vi "Main.vi"() -> ()   [LabVIEW 2015]
doc: "This template is for the Queued Message Handler design pattern.\n\nThe Event Handling Loop generates messages based on user interface actions.\n\nThe Message Handling Loop processes messages generated by the Event Handling Loop, or by other messages. The messages are string values, so new messages can be added easily to the Message Cases case structure in the Message Handling Loop. Each message cluster can also provide an optional value for Message Data, which is a variant that can be converted to whatever message-specific data is required."
uses:
  support/Type Definitions/UI Data.ctl
  support/Status Logger/Status Log.ctl
  <vilib>/Utility/error.llb/DialogType.ctl
  DAQ/TypeDefs/DAQ data.ctl
  support/Message Queue/Enqueue Message (Single).vi
  support/Global names.vi
  <vilib>/Utility/error.llb/Error Cluster From Error Code.vi
  <vilib>/ErrorRing/Error Ring.xnode
  support/Message Queue/Message Queue.lvlib
  support/User Event - EHL Stop/User Event - EHL Stop.lvlib
  Model/Model.lvlib
  DAQ/DAQ.lvlib
  PLC/PLC.lvlib
  Logger/Logger.lvlib
panel:
  out "Power status":bool
  in  "Remote":bool
  in  "Abort":bool
  in  "Stop Line":bool
  in  "Start Line":bool
  out "Status":string
  in  "Tab Control":T1(tab)
  in  "Power switch":bool
  in  "Positon":dbl(slide) scale=0.0..20.0
  in  "Dispose":bool
  in  "Pump":bool
  in  "Flow [l/s]":dbl=10.0
  in  "Potentiometer (AI)":tag
  in  "LED (DO)":tag
  in  "Bistable switch (DI)":tag
  in  "Monostable switch (DI)":tag
  in  "Send":bool
  in  "Data to send":string
  out "Data received":string
  in  "Disconnect":bool
  in  "Connect":bool
  out "Connected?":bool
  in  "Type":enum16{"Server", "Client"}(ring)
  in  "Port":u16
  in  "IP":string
  in  "Current printer":u16(ring) items=["PDFCreator", "OKI DATA CORP C5950 kolor (C-2 218)", "Microsoft XPS Document Writer", "Microsoft Print to PDF", "HP LaserJet Professional P1606dn B&W (M3)", "hp LaserJet 1320 PCL 5 B&W (C-2 307)", "Fax", "Canon MP560 KOLOR (DOM)", "Brother PC-FAX v.3.2", "Brother MFC-L8850CDW KOLOR (M6)", "Brother MFC-L2740DW B&W (M6)", "Brother MFC-L2740DW B&W (M3)", "Brother DCP-9020CDW (Dziekan)"]
  in  "Check printers":bool
  in  "Print report":bool
  in  "TDMS View":bool
  in  "Exit":bool
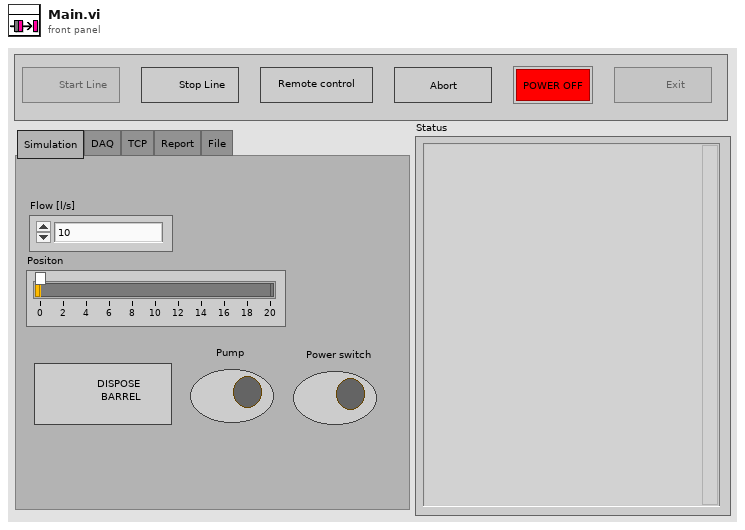
[diagram p1: front panel]
types:
  T1 = enum32{"Simulation", "DAQ", "TCP", "Report", "File"}
  T2 = typedef "Status Log.ctl" = enum16{"Close file", "Open Status file", "Add Status", "Show Status File"}
  T3 = typedef "UI Data.ctl" = cluster{"Start Line Ref":refnum<vi>, "Stop Line Ref":refnum<vi>, "Data Display Ref":refnum<vi>, "Exit Button Ref":refnum<vi>, "Pump Ref":refnum<vi>, "Dispose Ref":refnum<vi>, "Flow Ref":refnum<vi>, "Position Ref":refnum<vi>, "Tab Ref":refnum<vi>, "Print report":refnum<vi>, "Remote":refnum<vi>, "Connection status":refnum<vi>, "Abort":refnum<vi>, "Power status":refnum<vi>, "Power switch":refnum<vi>}
  T4 = typedef "Notifiers.lvlib/Notifiers.ctl" = cluster{"PLC":refnum<notifier>, "Model":refnum<notifier>, "DAQ":refnum<notifier>, "Log":refnum<notifier>}
  T5 = typedef "Message Queue.lvlib/All Message Queues.ctl" = cluster{"UI":refnum<queue>, "Model":refnum<queue>, "DAQ":refnum<queue>, "PLC":refnum<queue>, "Log":refnum<queue>}
  T6 = typedef "DialogType.ctl" = u16
  T7 = typedef "DAQ.lvlib/DAQ data.ctl" = cluster{"Power switch (DI)":cluster{"Channel":tag, "Data":bool}, "Dispose barrel (DI)":cluster{"Channel":tag, "Data":bool}, "Pump status (DO)":cluster{"Channel":tag, "Data":bool}, "Barrel position (AI)":cluster{"Channel":tag, "Data":dbl}}
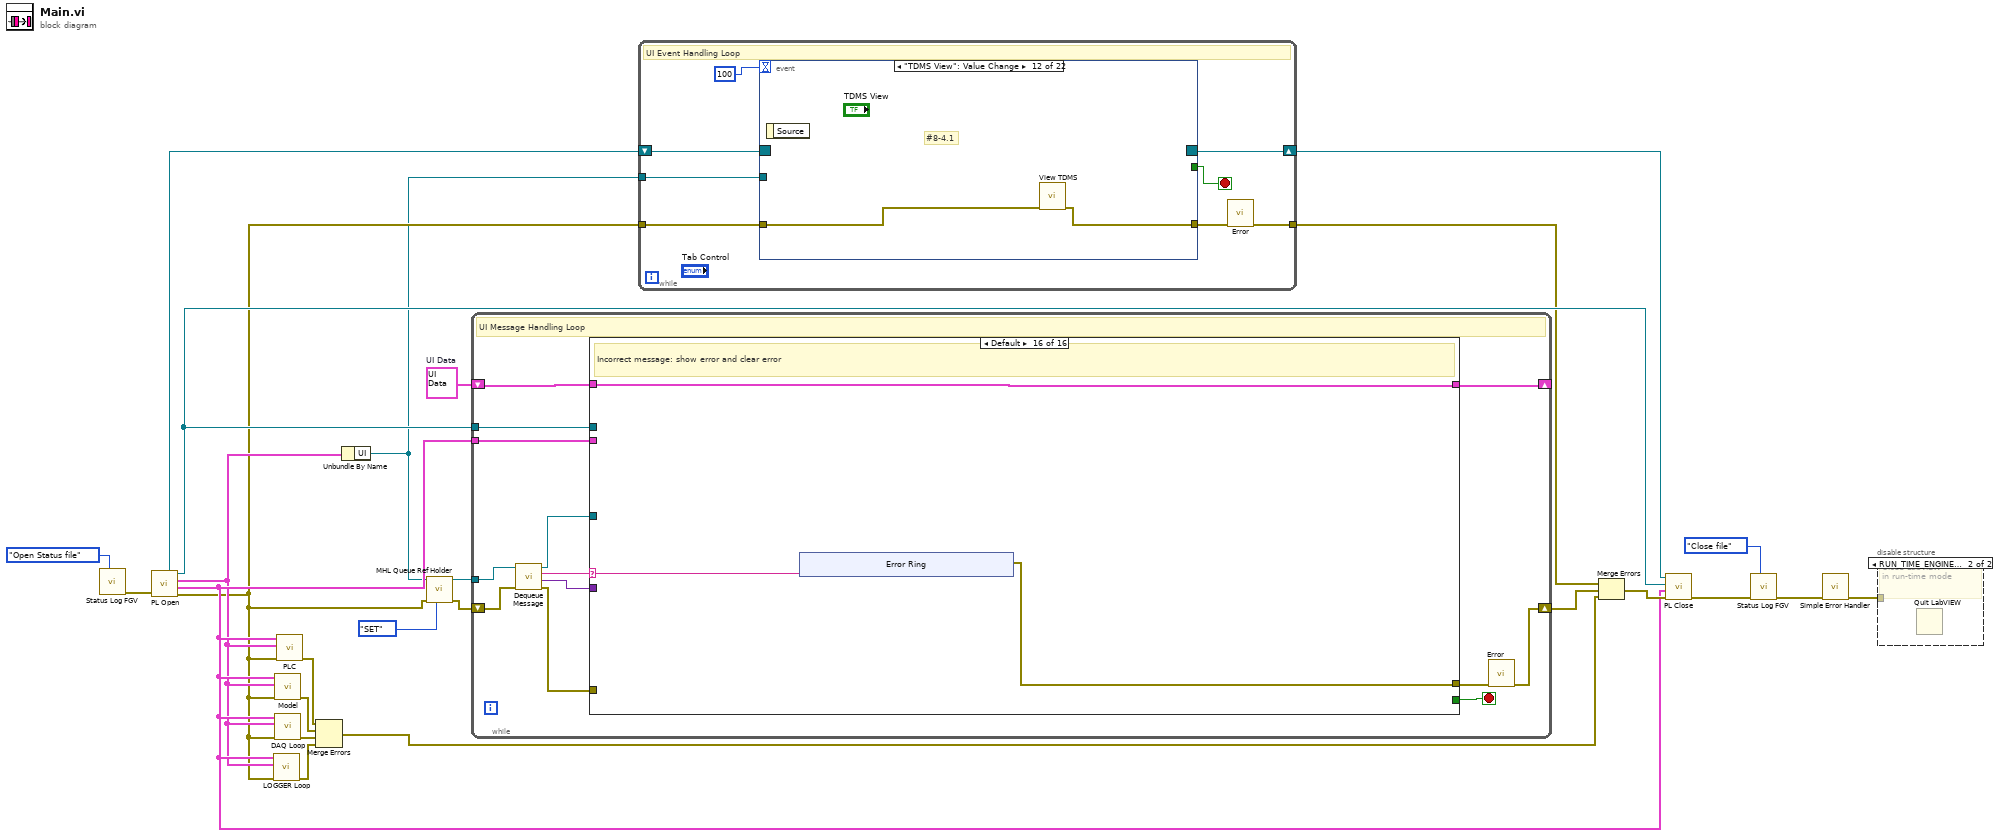
[diagram p0: block diagram]
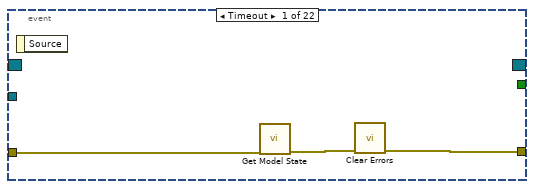
[diagram p2: hidden frame]
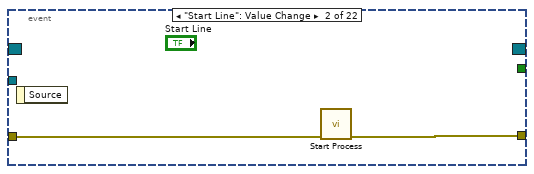
[diagram p3: hidden frame]
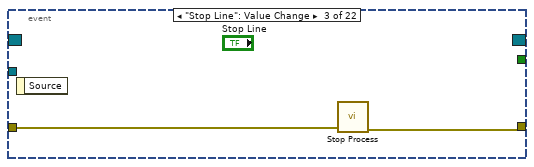
[diagram p4: hidden frame]
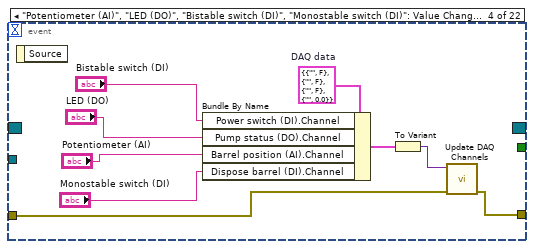
[diagram p5: hidden frame]
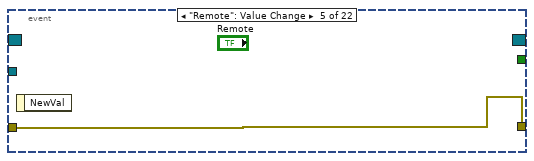
[diagram p6: hidden frame]
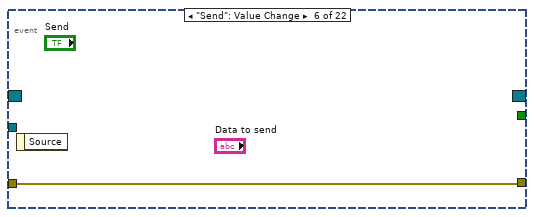
[diagram p7: hidden frame]
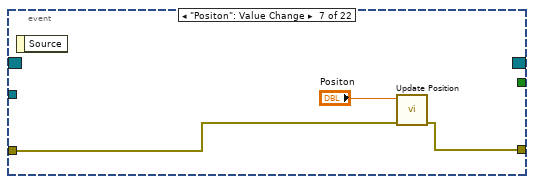
[diagram p8: hidden frame]
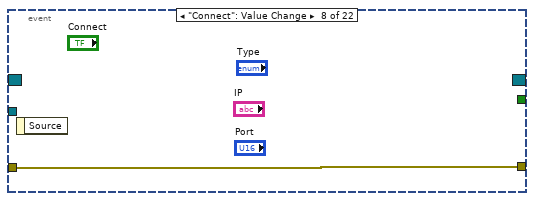
[diagram p9: hidden frame]
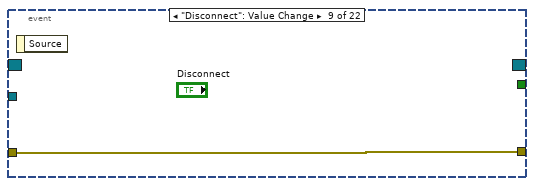
[diagram p10: hidden frame]
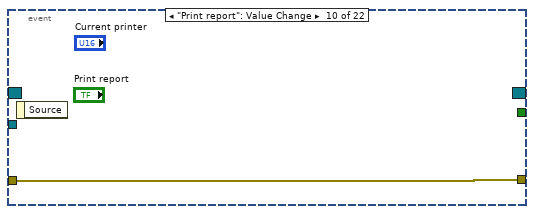
[diagram p11: hidden frame]
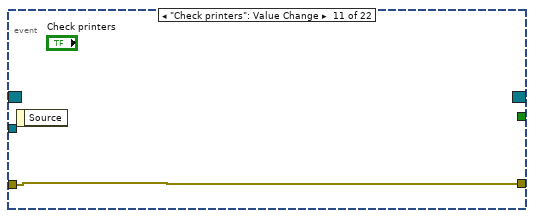
[diagram p12: hidden frame]
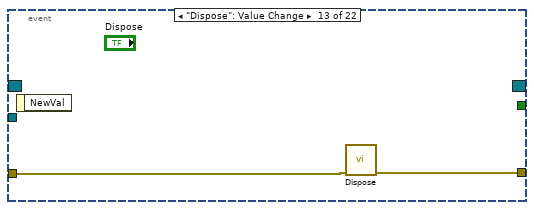
[diagram p13: hidden frame]
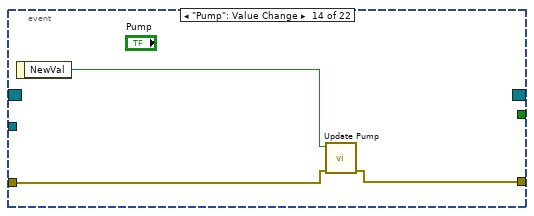
[diagram p14: hidden frame]
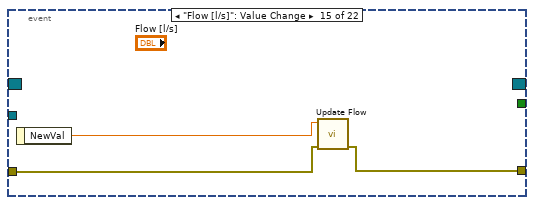
[diagram p15: hidden frame]
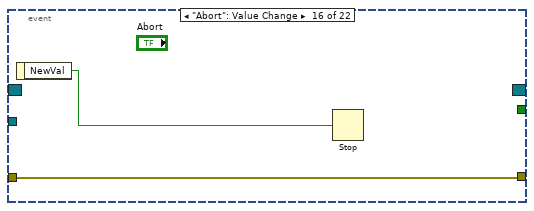
[diagram p16: hidden frame]
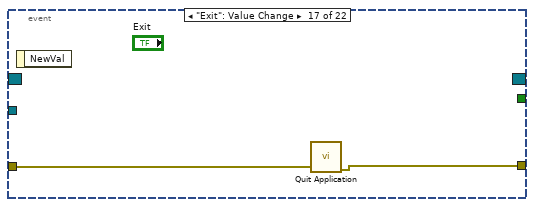
[diagram p17: hidden frame]
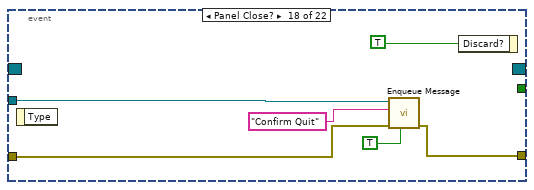
[diagram p18: hidden frame]
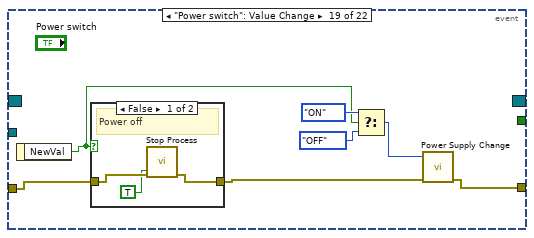
[diagram p19: hidden frame]
diagram:
  w24 = T3 {"Start Line Ref"=refnum, "Stop Line Ref"=refnum, "Data Display Ref"=refnum, "Exit Button Ref"=refnum, "Pump Ref"=refnum, "Dispose Ref"=refnum, "Flow Ref"=refnum, "Position Ref"=refnum, "Tab Ref"=refnum, "Print report"=refnum, "Remote"=refnum, "Connection status"=refnum, "Abort"=refnum, "Power status"=refnum, "Power switch"=refnum}  # UI Data
  n1 = call "Status Log FGV.vi"("Action"=Status_Log."Open Status file") -> ("error out"=w19:errorcluster)  [unwired: 10 in]
  n2 = call "PL Open.vi"("error in"=w19) -> ("error out"=w4:errorcluster, "Notifiers"=w12:T4, "Queues"=w11:T5, "User Event"=w22:refnum<user-event>, "Event Registration Refnum"=w14:refnum<event-registration>)  [unwired: 6 in]
  n3 = call "LOGGER Loop.vi"("error in"=w4, "Queues"=w11, "Notifiers"=w12) -> ("error out"=w7:errorcluster)  [unwired: 8 in]
  n4 = call "Model.vi"("error in"=w4, "Queues"=w11, "Notifiers"=w12) -> ("error out"=w9:errorcluster)  [unwired: 8 in]
  n5 = call "DAQ Loop.vi"("error in"=w4, "Queues"=w11, "Notifiers"=w12) -> ("error out"=w8:errorcluster)  [unwired: 8 in]
  n6 = call "PLC.vi"("error in"=w4, "Message Queues"=w11, "Notifiers"=w12) -> ("error out"=w10:errorcluster)  [unwired: 8 in]
  n7 = Merge Errors(w10, w9, w8, w7) -> (w6:errorcluster)
  n8 = Unbundle By Name(w11) -> ("UI"=w1:refnum<queue>)
  n9 = call "MHL Queue Ref Holder.vi"("Action"=enum16{"GET", "SET"}."SET", "error in"=w4, "Message Queue In"=w1) -> ("error out"=w3:errorcluster, "Input Message Queue"=w5:refnum<queue>)  [unwired: 7 in]
  n10 = while {
    shift-right: [w37] -> _
    shift-left: w24 -> [w38]
    tunnel: w22 -> [w35]
    tunnel: w12 -> [w31]
    shift-right: [w27] -> w18
    shift-left: w3 -> [w34]
    tunnel: w5 -> [w29]
    stop <- w36 stop-if-true
    # "UI Message Handling Loop"
    n11 = call "Dequeue Message.vi"("error in (no error)"=w34, "Message Queue"=w29) -> ("error out"=w33:errorcluster, "Message Data"=w30:variant, "Message"=w26:string, "dup Message Queue"=w32:refnum<queue>)  [unwired: 6 in]
    n12 = case "Message Cases" shown="Default" w26 {
      selector: w26 -> [_ _ _ _ _ _ _ _ _ _ _ _ _ _ _ w269]
      tunnel: w32 -> [w40 _ _ _ _ _ _ _ _ _ _ w215 w221 w257 _ _]
      tunnel: w33 -> [w41 w47 w70 w104 w119 w138 w152 w168 w175 w204 w207 w216 w223 w240 w264 _]
      tunnel: [w39 w47 w79 w105 w118 w140 w153 w169 w175 w200 w206 w213 w220 w244 w258 w268] -> w28
      tunnel: w38 -> [w42 w61 w90 w106 w125 w150 w159 w172 w176 w182 w211 w217 w227 w249 w263 w270]
      tunnel: [w42 w48 w90 w106 w125 w150 w159 w172 w176 w182 w211 w217 w227 w249 w263 w270] -> w37
      tunnel: [_ _ _ _ _ _ _ _ _ _ _ _ _ TRUE _ _] -> w36
      tunnel: w30 -> [_ _ _ _ _ _ w163 w166 _ w203 w210 _ _ w251 _ _]
      tunnel: w35 -> [_ _ _ _ _ _ _ _ _ _ _ _ _ w254 _ _]
      tunnel: w31 -> [_ _ _ _ _ _ _ _ _ _ _ _ w226 _ _ _]
      frame "Initialize" {
        w43 = string[] ["Initialize references", "Initialize controls", "Initialize PLC"]  # Message
        # "Prepare application initialization procedure"
        n13 = call "Enqueue Message (Array).vi"("error in (no error)"=w41, "Message Array"=w43, "Message Queue"=w40) -> ("error out"=w39:errorcluster)  [unwired: 7 in, 1 out]
      }
      frame "Initialize references" {
        # "Link references to UI objects"
        n14 = control-ref of="Power switch"() -> (w44:refnum<vi>)
        n15 = control-ref of="Stop Line"() -> (w58:refnum<vi>)
        n16 = control-ref of="Flow [l/s]"() -> (w55:refnum<vi>)
        n17 = control-ref of="Dispose"() -> (w56:refnum<vi>)
        n18 = control-ref of="Exit"() -> (w60:refnum<vi>)
        n19 = control-ref of="Start Line"() -> (w59:refnum<vi>)
        n20 = control-ref of="Pump"() -> (w57:refnum<vi>)
        n21 = Bundle By Name(cluster=w61, "Exit Button Ref"=w60, "Start Line Ref"=w59, "Stop Line Ref"=w58, "Pump Ref"=w57, "Dispose Ref"=w56, "Flow Ref"=w55, "Power switch"=w44) -> (w54:T3)
        n22 = control-ref of="Tab Control"() -> (w52:refnum<vi>)
        n23 = control-ref of="Remote"() -> (w50:refnum<vi>)
        n24 = control-ref of="Connection status"() -> (w49:refnum<vi>)
        n25 = control-ref of="Positon"() -> (w53:refnum<vi>)
        n26 = control-ref of="Print report"() -> (w51:refnum<vi>)
        n27 = control-ref of="Power status"() -> (w45:refnum<vi>)
        n28 = control-ref of="Abort"() -> (w46:refnum<vi>)
        n29 = Bundle By Name(cluster=w54, "Position Ref"=w53, "Tab Ref"=w52, "Print report"=w51, "Remote"=w50, "Connection status"=w49, "Abort"=w46, "Power status"=w45) -> (w48:T3)
      }
      frame "Initialize controls" {
        w62 = TRUE ("Enabled")
        w63 = FALSE ("Enabled")
        # "Initialize activity and values of UI objects"
        n30 = Unbundle By Name(w90) -> ("Stop Line Ref"=w103:refnum<vi>, "Print report"=w85:refnum<vi>)
        n31 = Current VI's Menubar() -> (w65:refnum<k9>)
        n32 = Build Array(w103, w85) -> (w102:refnum<vi>[])
        n33 = call "Enable Multiple Controls.vi"("error in"=w70, "Enabled"=w63, "References"=w102) -> ("error out"=w99:errorcluster)  [unwired: 8 in]
        n34 = Set Menu Item Info(7:"Stop" ("item tag"), 8:w70, 9:w63, 11:w65) -> (0:w68:errorcluster, 3:w64:refnum<k9>)  [unwired: 3 in]
        n35 = Unbundle By Name(w90) -> ("Exit Button Ref"=w101:refnum<vi>, "Start Line Ref"=w100:refnum<vi>)
        n36 = call "Power Supply Change.vi"("error in"=w70, "Power status"=enum16{"OFF", "ON"}."OFF") -> ("error out"=w76:errorcluster)  [unwired: 9 in]
        n37 = Build Array(w101, w100) -> (w98:refnum<vi>[])
        n38 = call "Enable Multiple Controls.vi"("error in"=w99, "Enabled"=w62, "References"=w98) -> ("error out"=w93:errorcluster)  [unwired: 8 in]
        n39 = Set Menu Item Info(7:"Start" ("item tag"), 8:w68, 9:w62, 11:w64) -> (0:w66:errorcluster)  [unwired: 3 in, 1 out]
        n40 = Unbundle By Name(w90) -> ("Exit Button Ref"=w97:refnum<vi>, "Start Line Ref"=w96:refnum<vi>, "Stop Line Ref"=w95:refnum<vi>, "Pump Ref"=w94:refnum<vi>, "Remote"=w84:refnum<vi>, "Connection status"=w83:refnum<vi>, "Abort"=w82:refnum<vi>, "Power status"=w81:refnum<vi>, "Power switch"=w72:refnum<vi>)
        n41 = call "Status Display.vi"("Action"=enum16{"Update", "Clear"}."Clear", "error in"=w76) -> ("error out"=w75:errorcluster, "Status"=w73:string)  [unwired: 8 in]
        n42 = local write "Status"(w73) -> ()
        n43 = Build Array(w97, w96, w95, w94, w84, w83, w82, w81, w72) -> (w91:refnum<vi>[])
        n44 = call "Value Multiple Boolean Controls.vi"("error in"=w93, "Value"=FALSE ("Enabled"), "References"=w91) -> ("error out"=w89:errorcluster)  [unwired: 8 in]
        n45 = Unbundle By Name(w90) -> ("Position Ref"=w88:refnum<vi>)
        n46 = Build Array(w88) -> (w87:refnum<vi>[])
        n47 = call "Value Multiple Numeric Controls.vi"("error in"=w89, "Value"=0.0, "References"=w87) -> ("error out"=w78:errorcluster)  [unwired: 8 in]
        n48 = call "Update Display.vi"("error in"=w78, "Message string"="UI initialized") -> ("error out"=w67:errorcluster)  [unwired: 9 in]
        n49 = Merge Errors(w67, w66, w75) -> (w79:errorcluster)
      }
      frame "Initialize PLC" {
        # "Initialize Production Line Controller"
        n50 = call "Initialize.vi"("error in"=w104) -> ("error out"=w105:errorcluster)  [unwired: 10 in]
      }
      frame "Start process" {
        w110 = TRUE ("Enabled")
        w114 = FALSE ("Enabled")
        # "Starts process: start PLC, open logger file, create reports files, enable/disable UI controls and update status display"
        n51 = Unbundle By Name(w125) -> ("Exit Button Ref"=w107:refnum<vi>, "Start Line Ref"=w120:refnum<vi>, "Stop Line Ref"=w124:refnum<vi>)
        n52 = Build Array(w107, w120) -> (w126:refnum<vi>[])
        n53 = Build Array(w124) -> (w123:refnum<vi>[])
        n54 = call "Start.vi"("error in"=w119) -> ("error out"=w122:errorcluster)  [unwired: 10 in]
        n55 = call "Enable Multiple Controls.vi"("error in"=w119, "Enabled"=w110, "References"=w123) -> ("error out"=w112:errorcluster)  [unwired: 8 in]
        n56 = call "Enable Multiple Controls.vi"("error in"=w119, "Enabled"=w114, "References"=w126) -> ("error out"=w116:errorcluster)  [unwired: 8 in]
        n57 = global read "Global names.vi" "Starting"() -> (w108:string)
        n58 = Current VI's Menubar() -> (w109:refnum<k9>)
        n59 = call "Update Display.vi"("error in"=w122, "Message string"=w108) -> ("error out"=w121:errorcluster)  [unwired: 9 in]
        n60 = Set Menu Item Info(7:"Start" ("item tag"), 8:w116, 9:w114, 11:w109) -> (0:w115:errorcluster)  [unwired: 3 in, 1 out]
        n61 = Set Menu Item Info(7:"Stop" ("item tag"), 8:w112, 9:w110, 11:w109) -> (0:w111:errorcluster)  [unwired: 3 in, 1 out]
        n62 = Merge Errors(w121, w115, w111) -> (w118:errorcluster)
      }
      frame "Stop process" {
        w129 = FALSE ("Enabled")
        w130 = TRUE ("Enabled")
        # "Stops process: stop PLC, close logger file, save and close report files, enable/disable UI controls and update status display"
        n63 = Unbundle By Name(w150) -> ("Exit Button Ref"=w127:refnum<vi>, "Start Line Ref"=w143:refnum<vi>, "Stop Line Ref"=w149:refnum<vi>)
        n64 = call "Stop.vi"("error in"=w138) -> ("error out"=w145:errorcluster)  [unwired: 10 in]
        n65 = Build Array(w149) -> (w139:refnum<vi>[])
        n66 = Build Array(w127, w143) -> (w147:refnum<vi>[])
        n67 = global read "Global names.vi" "Stopping"() -> (w128:string)
        n68 = Build Array (concatenate)(w147, w139) -> (w146:refnum<vi>[])
        n69 = call "Enable Multiple Controls.vi"("error in"=w138, "Enabled"=w130, "References"=w147) -> ("error out"=w135:errorcluster)  [unwired: 8 in]
        n70 = call "Enable Multiple Controls.vi"("error in"=w138, "Enabled"=w129, "References"=w139) -> ("error out"=w142:errorcluster)  [unwired: 8 in]
        n71 = call "Value Multiple Boolean Controls.vi"("error in"=w138, "Value"=FALSE, "References"=w146) -> ("error out"=w141:errorcluster)  [unwired: 8 in]
        n72 = call "Update Display.vi"("error in"=w145, "Message string"=w128) -> ("error out"=w144:errorcluster)  [unwired: 9 in]
        n73 = Current VI's Menubar() -> (w136:refnum<k9>)
        n74 = Set Menu Item Info(7:"Start" ("item tag"), 8:w135, 9:w130, 11:w136) -> (0:w133:errorcluster, 3:w131:refnum<k9>)  [unwired: 3 in]
        n75 = Set Menu Item Info(7:"Stop" ("item tag"), 8:w133, 9:w129, 11:w131) -> (0:w132:errorcluster)  [unwired: 3 in, 1 out]
        n76 = Merge Errors(w144, w132, w142, w141) -> (w140:errorcluster)
      }
      frame "Update display" {
        # "Updates status display, status log file and word report file"
        n77 = Variant To Data(error in=w152, type="", Variant=w163) -> (data=w151:string, error out=w156:errorcluster)
        n78 = call "Status Display.vi"("Action"=enum16{"Update", "Clear"}."Update", "error in"=w156, "Status line"=w151) -> ("error out"=w154:errorcluster, "Status"=→"Status":string)  [unwired: 7 in]
        n79 = call "Status Log FGV.vi"("Action"=Status_Log."Add Status", "error in"=w156, "Status"=w151) -> ("error out"=w155:errorcluster)  [unwired: 8 in]
        n80 = property on="Status" class="Str"("Text.Scroll Position"=-1) -> ()  [unwired: 2 in, 2 out]
        n81 = Merge Errors(w155, w154) -> (w153:errorcluster)
      }
      frame "Update position" {
        # "Programmatically update position of the barrel slider"
        n82 = Variant To Data(error in=w168, type=0.0 ("Value"), Variant=w166) -> (data=w164:dbl, error out=w167:errorcluster)
        n83 = Unbundle By Name(w172) -> ("Position Ref"=w171:refnum<vi>)
        n84 = Build Array(w171) -> (w170:refnum<vi>[])
        n85 = call "Value Multiple Numeric Controls.vi"("error in"=w167, "Value"=w164, "References"=w170) -> ("error out"=w169:errorcluster)  [unwired: 8 in]
      }
      frame "Update Connection UI" {
        # "Updates TCP conection UI indicators"
        "Data received" <- "" ("Data received")
        "Connected?" <- FALSE ("Connected?")
      }
      frame "Power status change" {
        # "Update main switch LED and Start/Stop buttons according to power status change (DAQ DI)"
        n86 = Variant To Data(error in=w204, type=TRUE, Variant=w203) -> (data=w183:bool, error out=w187:errorcluster)
        "Power status" <- w183
        n87 = Unbundle By Name(w182) -> ("Position Ref"=w177:refnum<vi>, "Dispose Ref"=w181:refnum<vi>, "Pump Ref"=w180:refnum<vi>)
        n88 = Unbundle By Name(w182) -> ("Start Line Ref"=w179:refnum<vi>, "Stop Line Ref"=w201:refnum<vi>)
        n89 = Build Array(w177, w181, w180, w179) -> (w178:refnum<vi>[])
        n90 = Build Array(w179) -> (w199:refnum<vi>[])
        n91 = Build Array(w201) -> (w196:refnum<vi>[])
        n92 = Build Array (concatenate)(w199, w196) -> (w198:refnum<vi>[])
        n93 = Current VI's Menubar() -> (w190:refnum<k9>)
        n94 = call "Enable Multiple Controls.vi"("error in"=w187, "Enabled"=w183, "References"=w178) -> ("error out"=w194:errorcluster)  [unwired: 8 in]
        n95 = Set Menu Item Info(7:"Start" ("item tag"), 8:w187, 9:w183, 11:w190) -> (0:w188:errorcluster, 3:w184:refnum<k9>)  [unwired: 3 in]
        n96 = call "Value Multiple Boolean Controls.vi"("error in"=w187, "Value"=FALSE, "References"=w198) -> ("error out"=w193:errorcluster)  [unwired: 8 in]
        n97 = call "Enable Multiple Controls.vi"("error in"=w187, "Enabled"=FALSE, "References"=w196) -> ("error out"=w192:errorcluster)  [unwired: 8 in]
        n98 = Set Menu Item Info(7:"Stop" ("item tag"), 8:w188, 9:FALSE ("enabled"), 11:w184) -> (0:w185:errorcluster)  [unwired: 3 in, 1 out]
        n99 = Merge Errors(w194, w193, w192, w185) -> (w200:errorcluster)
      }
      frame "Error" {
        w205 = T6 2 items=["no dialog", "OK message", "continue or stop message", "OK message + warnings", "continue/stop + warnings"] ("type of dialog (OK msg:1)")
        # "Display error dialog box and quit application"
        n100 = Variant To Data(error in=w207, type=errorcluster {"status"=FALSE, "code"=0, "source"=""} ("error constant"), Variant=w210) -> (data=w208:errorcluster, error out=w206:errorcluster)
        n101 = call <vilib>:"Simple Error Handler.vi"("type of dialog (OK msg:1)"=w205, "error in (no error)"=w208) -> ()  [unwired: 3 in, 5 out]
      }
      frame "Exit" {
        # "Start exit procedure: stop PLC, then send Exit message to PLC and go to PLC confirmation loop"
        n102 = Flush Queue(queue=w215, error in (no error)=w216) -> (error out=w212:errorcluster)  [unwired: 2 out]
        n103 = call "Exit PLC.vi"("error in"=w212) -> ("error out"=w214:errorcluster)  [unwired: 10 in]
        n104 = call "Wait on PLC Exit.vi"("error in"=w214) -> ("error out"=w213:errorcluster)  [unwired: 10 in]
      }
      frame "Wait on PLC exit" {
        # "Wait until PLC shutdown"
        n105 = Unbundle By Name(w226) -> ("PLC"=w225:refnum<notifier>)
        n106 = Wait on Notification(notifier=w225, timeout in ms (-1)=10, error in (no error)=w223) -> (notification=w219:string, timed out?=w222:bool, error out=w218:errorcluster)  [unwired: 1 in, 1 out]
        n107 = case shown="True" w222 {
          tunnel: [w228 w237] -> w220
          tunnel: w218 -> [w229 w234]
          tunnel: w221 -> [_ w235]
          tunnel: w219 -> [_ w230]
          frame True {
            # "Shutdown notification from PLC not received"
            n108 = call "Wait on PLC Exit.vi"("error in"=w229) -> ("error out"=w228:errorcluster)  [unwired: 10 in]
          }
          frame False {
            # "Shutdown notification from PLC received (handshake)"
            n109 = call "Update Display.vi"("error in"=w234, "Message string"=w230) -> ("error out"=w233:errorcluster)  [unwired: 9 in]
            n110 = call "Update Display.vi"("error in"=w233, "Message string"="Application quits" ("Message")) -> ("error out"=w232:errorcluster)  [unwired: 9 in]
            n111 = call-poly "Enqueue Message.vi"("error in (no error)"=w232, "Message"="End program", "Message Queue"=w235) -> ("error out"=w237:errorcluster)  [unwired: 7 in, 1 out]
          }
        }
      }
      frame "End program" {
        # "Shutdown MHL and send exit user event to EHL; reset UI controls"
        n112 = call "Fire User Event - EHL Stop.vi"("error in (no error)"=w240, "User Event - Stop"=w254) -> ("error out"=w239:errorcluster)  [unwired: 9 in]
        n113 = Variant To Data(error in=w240, type=errorcluster {"status"=FALSE, "code"=0, "source"=""} ("error constant"), Variant=w251) -> (data=w252:errorcluster)  [unwired: 1 out]
        n114 = Release Queue(queue=w257, force destroy? (F)=TRUE, error in (no error)=w240) -> (error out=w255:errorcluster)  [unwired: 2 out]
        n115 = call <vilib>:"Simple Error Handler.vi"("error in (no error)"=w252) -> ("error out"=w238:errorcluster)  [unwired: 4 in, 4 out]
        n116 = Merge Errors(w239, w238, w255) -> (w245:errorcluster)
        n117 = Unbundle By Name(w249) -> ("Exit Button Ref"=w248:refnum<vi>, "Abort"=w243:refnum<vi>, "Start Line Ref"=w242:refnum<vi>, "Stop Line Ref"=w241:refnum<vi>)
        n118 = Build Array(w248, w243, w242, w241) -> (w247:refnum<vi>[])
        n119 = call "Value Multiple Boolean Controls.vi"("error in"=w245, "Value"=FALSE, "References"=w247) -> ("error out"=w244:errorcluster)  [unwired: 8 in]
      }
      frame "Confirm Quit" {
        # "Confirm Quit - Message that can confirm whether or not the user wants to exit the application."
        n120 = Two Button Dialog(message="Are you sure?", 1:"Continue" ("F button name (\"Cancel\")"), 2:"Quit" ("T button name (\"OK\")")) -> (T button?=w259:bool)
        n121 = case shown="True" w259 {
          tunnel: w264 -> [w265 w267]
          tunnel: [w265 w266] -> w258
          frame False {
          }
          frame True {
            n122 = call "Quit Application.vi"("error in"=w267) -> ("error out"=w266:errorcluster)  [unwired: 10 in]
          }
        }
      }
      frame Default {
        # "Incorrect message: show error and clear error"
        n123 = xnode "Error Ring"("parameter 0"=w269) -> ("error out"=w268:errorcluster)
      }
    }
    n124 = call "Error.vi"("error in"=w28) -> ("error out"=w27:errorcluster)  [unwired: 10 in]
  }
  n125 = while {
    tunnel: w1 -> [w280]
    shift-right: [w284] -> w25
    shift-left: w14 -> [w285]
    tunnel: [w278] -> w13
    tunnel: w4 -> [w281]
    stop <- w283 stop-if-true
    # "UI Event Handling Loop"
    n126 = event shown="[11] \"TDMS View\": Value Change" {
      selector: w285 -> [_ _ _ _ _ _ _ _ _ _ _ _ _ _ _ _ _ _ _ _ _ _]
      dyn-events: [_ _ _ _ _ _ _ _ _ _ _ _ _ _ _ _ _ _ _ _ _ _] -> w284
      timeout: 100 -> [_ _ _ _ _ _ _ _ _ _ _ _ _ _ _ _ _ _ _ _ _ _]
      tunnel: [_ _ _ _ _ _ _ _ _ _ _ _ _ _ _ _ _ _ _ _ TRUE ("Discard?") _] -> w283
      tunnel: w280 -> [_ _ _ _ _ _ _ _ _ _ _ _ _ _ _ _ _ w330 _ _ _ _]
      tunnel: [w286 w289 w291 w301 w302 w303 w305 w307 w308 w309 w310 w311 w313 w316 w319 w322 w323 w329 w331 w342 w343 w346] -> w279
      tunnel: w281 -> [w288 w290 w292 w300 w302 w303 w304 w307 w308 w309 w310 w312 w314 w317 w320 w322 w324 w325 w333 w342 w343 w345]
      event Timeout {
        n127 = event-data() -> ()  [unwired: 1 in, 1 out]
        n128 = call "Get Model State.vi"("error in (no error)"=w288) -> ("error out"=w287:errorcluster)  [unwired: 10 in]
        n129 = call <vilib>:"Clear Errors.vi"("error in (no error)"=w287) -> ("error out"=w286:errorcluster)  [unwired: 5 in, 1 out]
      }
      event "Start Line": Value Change {
        n130 = event-data() -> ()  [unwired: 1 in, 1 out]
        n131 = call "Start Process.vi"("error in"=w290) -> ("error out"=w289:errorcluster)  [unwired: 10 in]
      }
      event "Stop Line": Value Change {
        n132 = event-data() -> ()  [unwired: 1 in, 1 out]
        n133 = call "Stop Process.vi"("error in"=w292) -> ("error out"=w291:errorcluster)  [unwired: 10 in]
      }
      event "Potentiometer (AI)", "LED (DO)", "Bistable switch (DI)", "Monostable switch (DI)": Value Change {
        w294 = T7 {"Power switch (DI)"={"Channel"="", "Data"=FALSE}, "Dispose barrel (DI)"={"Channel"="", "Data"=FALSE}, "Pump status (DO)"={"Channel"="", "Data"=FALSE}, "Barrel position (AI)"={"Channel"="", "Data"=0.0}}  # DAQ data
        n134 = event-data() -> ()  [unwired: 1 in, 1 out]
        n135 = Bundle By Name(cluster=w294, "Power switch (DI).Channel"="Bistable switch (DI)", "Pump status (DO).Channel"="LED (DO)", "Barrel position (AI).Channel"="Potentiometer (AI)", "Dispose barrel (DI).Channel"="Monostable switch (DI)") -> (w297:T7)
        n136 = To Variant(anything=w297) -> (Variant=w293:variant)
        n137 = call "Update DAQ Channels.vi"("error in"=w300, "Message Data"=w293) -> ("error out"=w301:errorcluster)  [unwired: 9 in]
      }
      event "Remote": Value Change {
        n138 = event-data() -> ()  [unwired: 1 in, 1 out]
      }
      event "Send": Value Change {
        n139 = event-data() -> ()  [unwired: 1 in, 1 out]
      }
      event "Positon": Value Change {
        n140 = event-data() -> ()  [unwired: 1 in, 1 out]
        n141 = call "Update Position.vi"("error in (no error)"=w304, "Position"="Positon") -> ("error out"=w305:errorcluster)  [unwired: 9 in]
      }
      event "Connect": Value Change {
        n142 = event-data() -> ()  [unwired: 1 in, 1 out]
      }
      event "Disconnect": Value Change {
        n143 = event-data() -> ()  [unwired: 1 in, 1 out]
      }
      event "Print report": Value Change {
        n144 = event-data() -> ()  [unwired: 1 in, 1 out]
      }
      event "Check printers": Value Change {
        n145 = event-data() -> ()  [unwired: 1 in, 1 out]
      }
      event "TDMS View": Value Change {
        # "#8-4.1"
        n146 = event-data() -> ()  [unwired: 1 in, 1 out]
        n147 = call "View TDMS.vi"("error in"=w312) -> ("error out"=w311:errorcluster)  [unwired: 10 in]
      }
      event "Dispose": Value Change {
        n148 = event-data() -> ()  [unwired: 1 in, 1 out]
        n149 = call "Dispose.vi"("error in (no error)"=w314) -> ("error out"=w313:errorcluster)  [unwired: 10 in]
      }
      event "Pump": Value Change {
        n150 = event-data() -> ("NewVal"=w315:bool)  [unwired: 1 in]
        n151 = call "Update Pump.vi"("error in (no error)"=w317, "Pump State"=w315) -> ("error out"=w316:errorcluster)  [unwired: 9 in]
      }
      event "Flow [l/s]": Value Change {
        n152 = event-data() -> ("NewVal"=w318:dbl)  [unwired: 1 in]
        n153 = call "Update Flow.vi"("error in (no error)"=w320, "Flow"=w318) -> ("error out"=w319:errorcluster)  [unwired: 9 in]
      }
      event "Abort": Value Change {
        n154 = event-data() -> ("NewVal"=w321:bool)  [unwired: 1 in]
        n155 = Stop(stop? (T)=w321) -> ()
      }
      event "Exit": Value Change {
        n156 = event-data() -> ()  [unwired: 1 in, 1 out]
        n157 = call "Quit Application.vi"("error in"=w324) -> ("error out"=w323:errorcluster)  [unwired: 10 in]
      }
      event Panel Close? {
        n158 = event-data() -> ()  [unwired: 1 in, 1 out]
        n159 = call-poly "Enqueue Message.vi"("Priority Message? (F)"=TRUE, "error in (no error)"=w325, "Message"="Confirm Quit", "Message Queue"=w330) -> ("error out"=w329:errorcluster)  [unwired: 6 in, 1 out]
        n160 = event-data("Discard?"=TRUE) -> ()  [unwired: 1 in, 1 out]
      }
      event "Power switch": Value Change {
        n161 = event-data() -> ("NewVal"=w334:bool)  [unwired: 1 in]
        n162 = case shown="False" w334 {
          tunnel: w333 -> [w340 w341]
          tunnel: [w339 w341] -> w332
          frame False {
            # "Power off"
            n163 = call "Stop Process.vi"("Priority Message? (F)"=TRUE, "error in"=w340) -> ("error out"=w339:errorcluster)  [unwired: 9 in]
          }
          frame True {
            # "Power on"
          }
        }
        n164 = Select(t=enum16{"OFF", "ON"}."ON" ("Power status"), s=w334, f=enum16{"OFF", "ON"}."OFF" ("Power status")) -> (s? t:f=w335:enum16{"OFF", "ON"})
        n165 = call "Power Supply Change.vi"("error in"=w332, "Power status"=w335) -> ("error out"=w331:errorcluster)  [unwired: 9 in]
      }
      event Application Instance Close {
        n166 = event-data() -> ()  [unwired: 1 in, 1 out]
      }
      event User Event {
        n167 = event-data() -> ()  [unwired: 1 in, 1 out]
      }
      event Menu Selection (User) {
        n168 = event-data() -> ("ItemTag"=w347:string)  [unwired: 1 in]
        n169 = case shown="\"statuslog\"" w347 {
          tunnel: [w348 w351 w352 w356 w357 w359] -> w346
          tunnel: w345 -> [w348 w350 w353 w355 w358 w360]
          frame Default {
          }
          frame "logdir" {
            n170 = global read "Global names.vi" "Status log dir"() -> (w349:string)
            n171 = call "Open Dir.vi"("error in"=w350, "dir"=w349) -> ("error out"=w351:errorcluster)  [unwired: 9 in]
          }
          frame "statuslog" {
            n172 = call "Status Log FGV.vi"("Action"=Status_Log."Show Status File", "error in"=w353) -> ("error out"=w352:errorcluster)  [unwired: 9 in]
          }
          frame "Start" {
            n173 = call "Start Process.vi"("error in"=w355) -> ("error out"=w356:errorcluster)  [unwired: 10 in]
          }
          frame "Stop" {
            n174 = call "Stop Process.vi"("error in"=w358) -> ("error out"=w357:errorcluster)  [unwired: 10 in]
          }
          frame "Exit" {
            n175 = call "Quit Application.vi"("error in"=w360) -> ("error out"=w359:errorcluster)  [unwired: 10 in]
          }
        }
      }
    }
    n176 = call "Error.vi"("error in"=w279) -> ("error out"=w278:errorcluster)  [unwired: 10 in]
  }
  n177 = Merge Errors(w13, w18, w6) -> (w17:errorcluster)
  n178 = call "PL Close.vi"("error in"=w17, "Notifiers"=w12, "User Event"=w22, "Event Registration Refnum in"=w25) -> ("error out"=w23:errorcluster)  [unwired: 7 in]
  n179 = call "Status Log FGV.vi"("Action"=Status_Log."Close file", "error in"=w23) -> ("error out"=w15:errorcluster)  [unwired: 9 in]
  n180 = call <vilib>:"Simple Error Handler.vi"("error in (no error)"=w15) -> ("error out"=w16:errorcluster)  [unwired: 4 in, 4 out]
  n181 = disable-structure shown="RUN_TIME_ENGINE==True" {
    disable-tunnel: w16 -> [_ _]
    frame condition #0 (active) {
    }
    frame condition #1 {
      # "Close LabVIEW\nin run-time mode"
      n182 = Quit LabVIEW() -> ()  [unwired: 1 in]
    }
  }
